vi "Observer.vi"(11 "Name (\"\" to Use UUID)":string) -> ()   [LabVIEW 2025]
uses:
  67f8aefd-9a70-417d-a373-caed4e92e9c8.vi
  acccbc90-5136-4eb0-8ada-bd77d99bf855.vi
  <userlib>/_NEVSTOP/Communicable State Machine(CSM)/AdvanceAPI/CSM - Revert Arguments-Safe String.vi
  <userlib>/_NEVSTOP/Communicable State Machine(CSM)/AdvanceAPI/CSM - Make String Arguments Safe.vi
  <userlib>/_NEVSTOP/Communicable State Machine(CSM)/AdvanceAPI/CSM - Break Down Multiple States String.vi
  <userlib>/_NEVSTOP/Communicable State Machine(CSM)/AdvanceAPI/CSM - Compact Multiple States.vi
  <userlib>/_NEVSTOP/Communicable State Machine(CSM)/AdvanceAPI/CSM - Keywords.vi
  <userlib>/_NEVSTOP/Communicable State Machine(CSM)/_Shared/Trim Single-line Text.vi
  <userlib>/_NEVSTOP/Communicable State Machine(CSM)/_Polymophic/Build Status Broadcast Message.vi
  <userlib>/_NEVSTOP/Communicable State Machine(CSM)/addons/MassData-Parameter/_support/FGV-MassData(lvlibp).vi
  <userlib>/_NEVSTOP/Communicable State Machine(CSM)/_Polymophic/Build Asynchronous Message with Arguments.vi
  <userlib>/_NEVSTOP/Communicable State Machine(CSM)/_Polymophic/Build Synchronous Message with Arguments.vi
  <userlib>/_NEVSTOP/Communicable State Machine(CSM)/Communicable State Machine.lvlib
panel:
  out "Error Occurred":errorcluster
  out "State History":string
  in  "Exit":bool
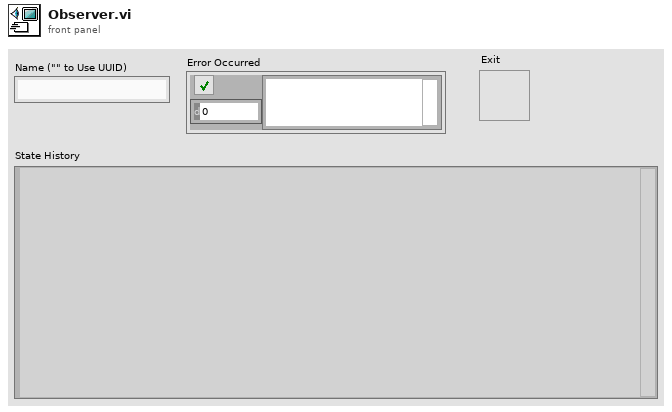
[diagram p1: front panel]
types:
  T1 = enum32{"Invalid", "Standard", "Closed", "Hidden", "Minimized", "Maximized"}
  T2 = enum32{"invalid app kind", "Development System", "Run Time System", "Student Edition", "Embedded LabVIEW", "Evaluation", "Custom"}
  T3 = typedef "Communicable State Machine.lvlib/_CSM_Response Source Message.ctl" = cluster{"‘State":string, "’Arguments":string, "’Error":errorcluster}
  T4 = cluster{"Current VI Reference":refnum<vi>, "Close Panel on Exit?":bool}
  T5 = cluster{"Core":cluster{"Current VI Reference":refnum<vi>, "Close Panel on Exit?":bool}, "player":cluster{"left":i16, "top":i16, "right":i16, "bottom":i16}, "step":i16, "Gate Condition":bool[]}
  T6 = cluster{"left":i16, "top":i16, "right":i16, "bottom":i16}
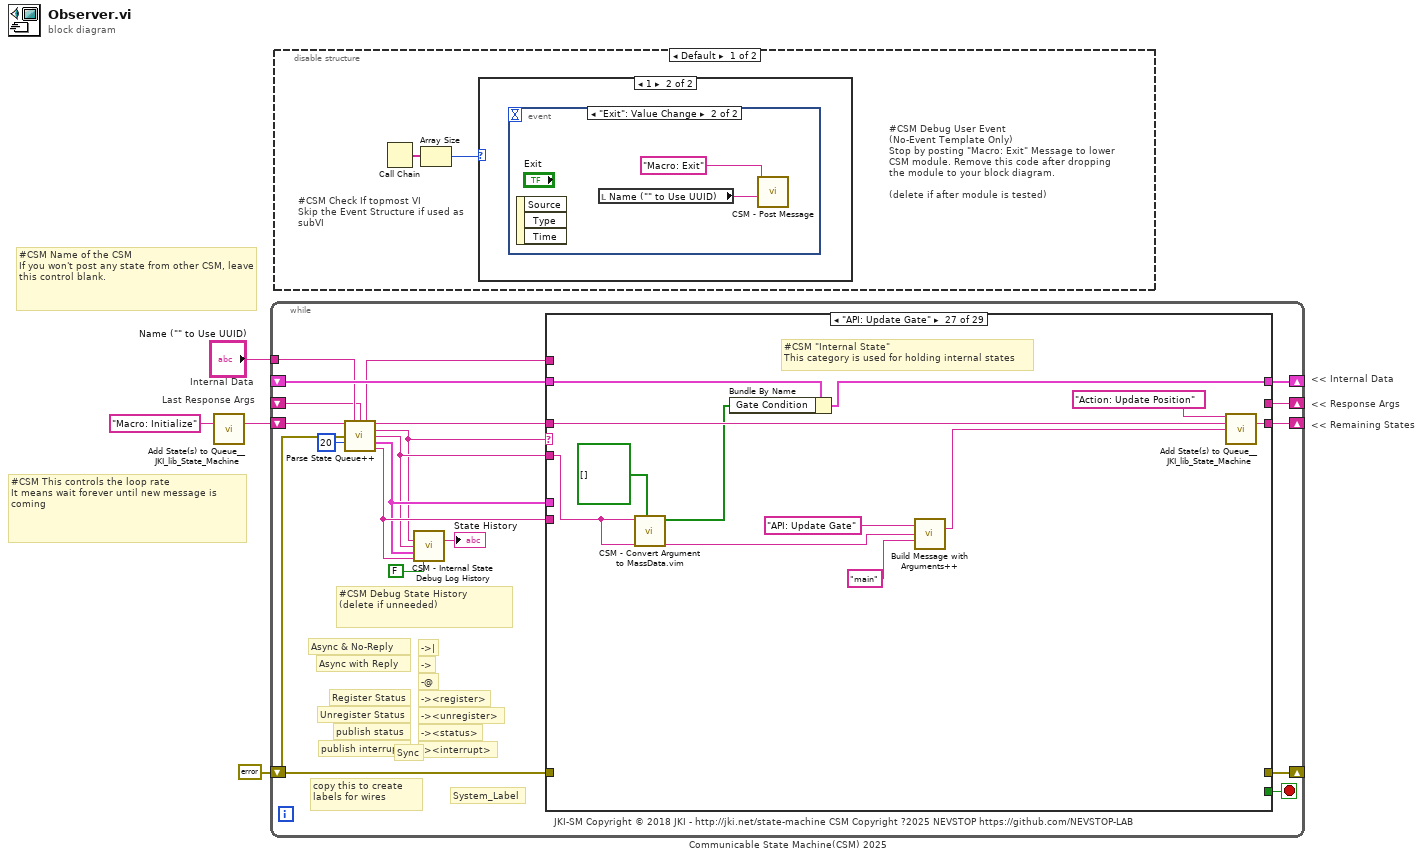
[diagram p0: block diagram]
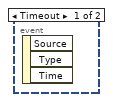
[diagram p3: hidden frame]
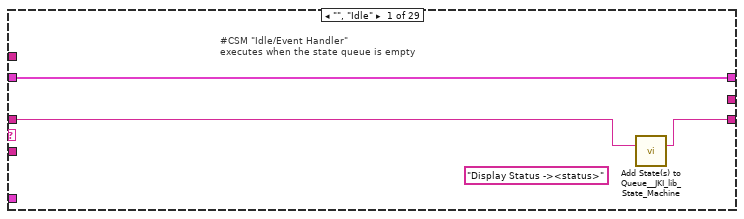
[diagram p5: hidden frame]
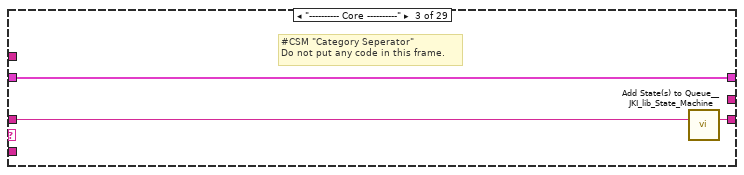
[diagram p7: hidden frame]
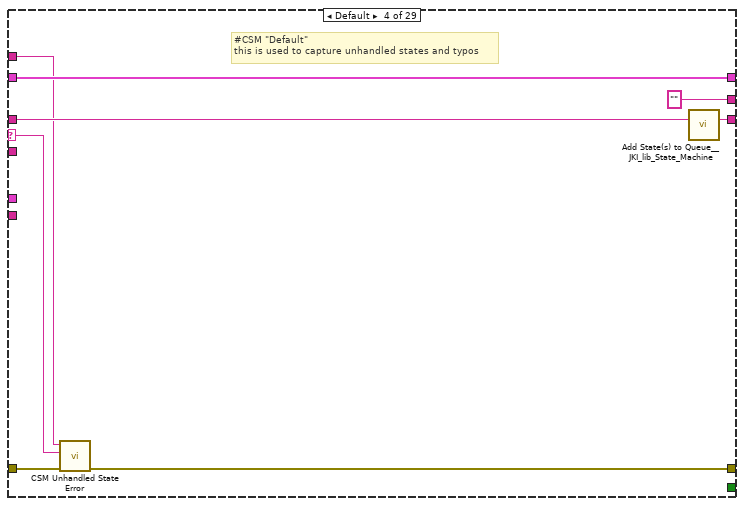
[diagram p8: hidden frame]
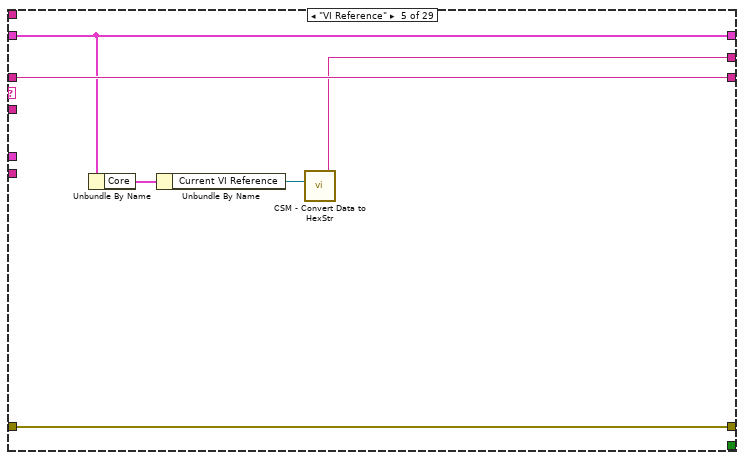
[diagram p9: hidden frame]
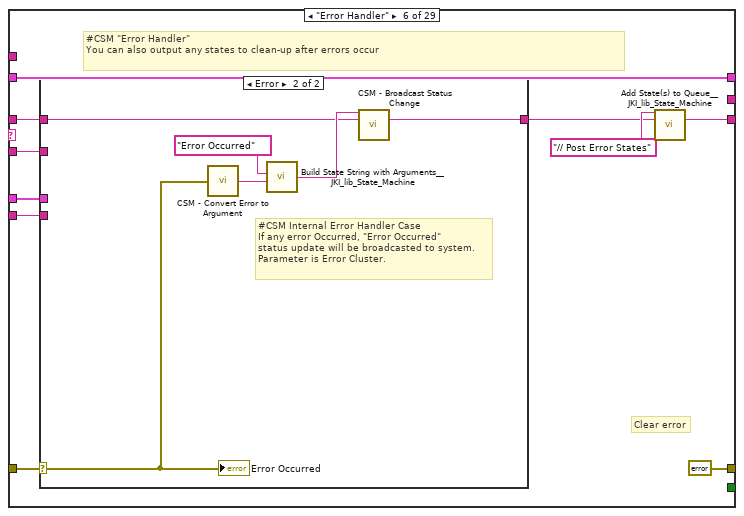
[diagram p10: hidden frame]
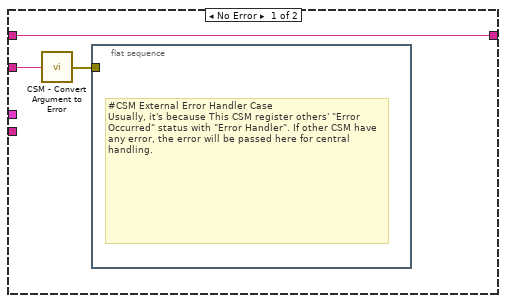
[diagram p11: hidden frame]
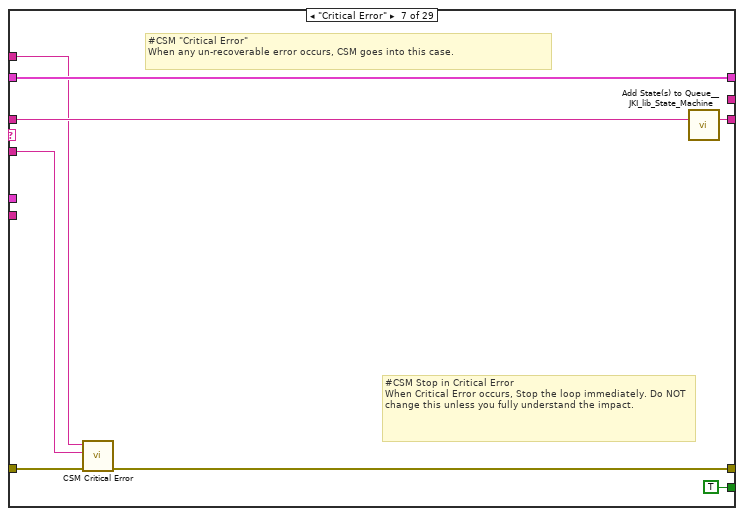
[diagram p12: hidden frame]
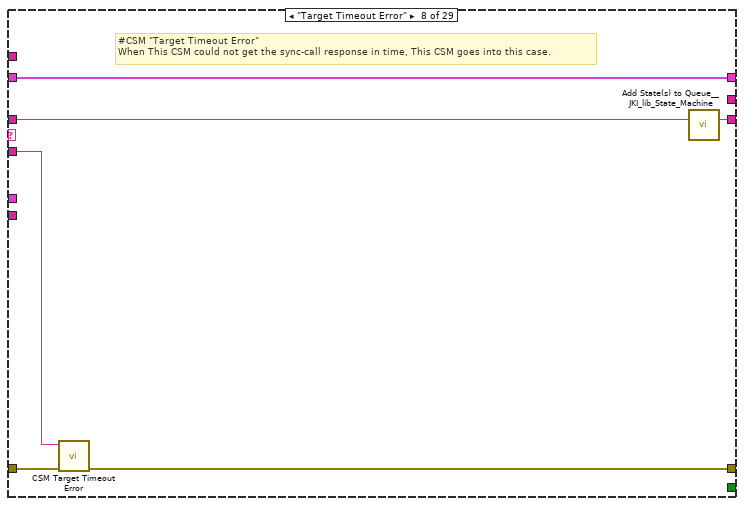
[diagram p13: hidden frame]
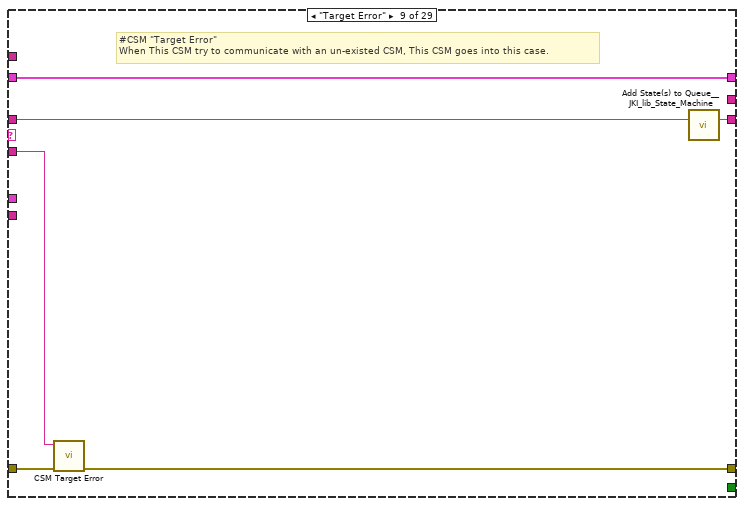
[diagram p14: hidden frame]
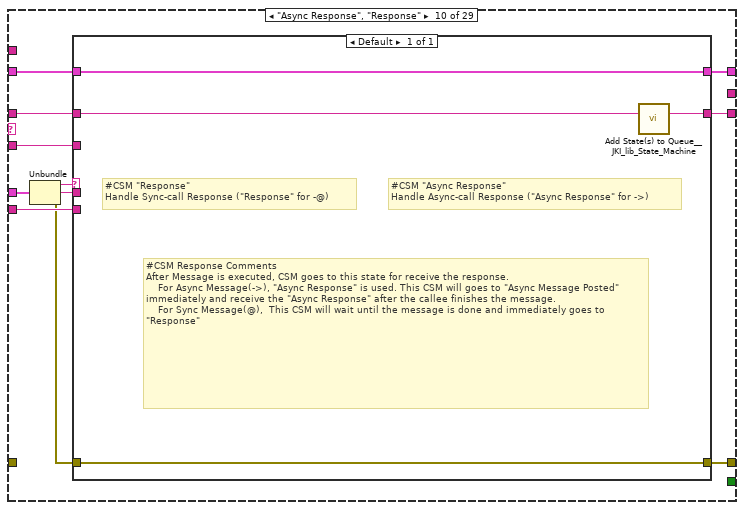
[diagram p15: hidden frame]
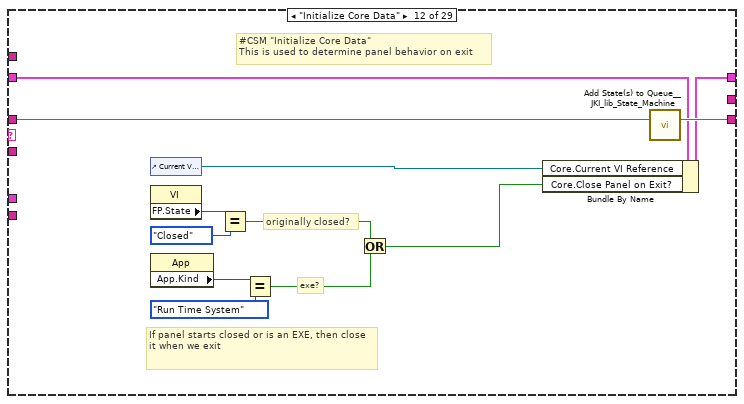
[diagram p17: hidden frame]
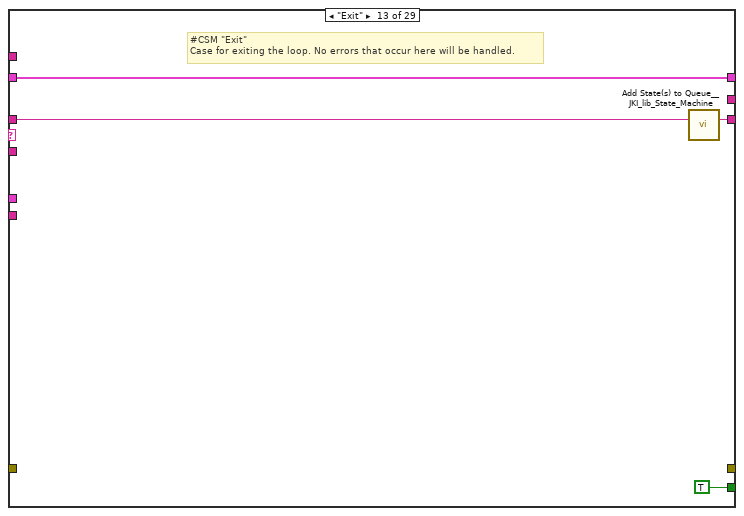
[diagram p18: hidden frame]
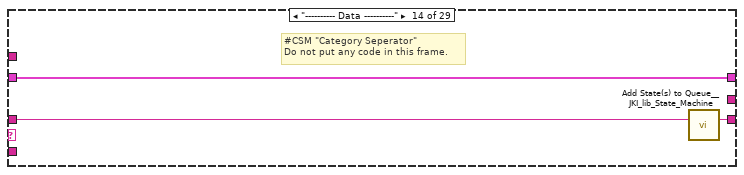
[diagram p19: hidden frame]
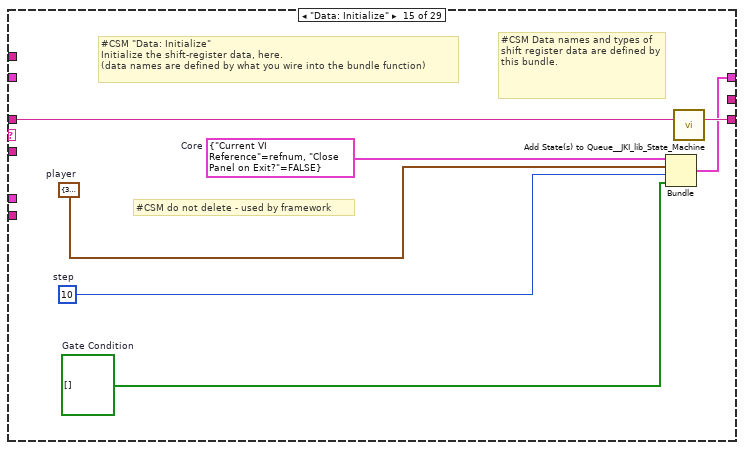
[diagram p20: hidden frame]
diagram:
  # "Last Response Args"
  # "Internal Data"
  # "#CSM Name of the CSM\nIf you won't post any state from other CSM, leave this control blank."
  # "#CSM This controls the loop rate\nIt means wait forever until new message is coming"
  # "<< Internal Data"
  # "<< Response Args"
  # "<< Remaining States"
  n1 = call <vilib>:"Add State(s) to Queue__JKI_lib_State_Machine.vi"("State(s) in (\"\")"="Macro: Initialize" ("Init State(\"Macro: Initialize\")")) -> ("States Out"=w1:string)  [unwired: 14 in]
  n2 = while "Communicable State Machine(CSM) 2025" {
    shift-right: [w18] -> _
    shift-left: _ -> [w17]
    shift-right: [w21] -> _
    shift-left: errorcluster {"status"=FALSE, "code"=0, "source"=""} ("error out") -> [w8]
    shift-right: [w20] -> _
    shift-left: w1 -> [w22]
    tunnel: "Name (\"\" to Use UUID)" -> [w15]
    shift-right: [w16] -> _
    shift-left: _ -> [w10]
    stop <- w19 stop-if-true
    # "#CSM Debug State History\n(delete if unneeded)"
    # "-><interrupt>"
    # "-><status>"
    # "-><unregister>"
    # "-><register>"
    # "-@"
    # "->"
    # "->|"
    # "publish interrupt"
    # "publish status"
    # "Unregister Status"
    # "Register Status"
    # "Sync"
    # "Async with Reply"
    # "Async & No-Reply"
    # "JKI-SM Copyright © 2018 JKI - http://jki.net/state-machine CSM Copyright ?2025 NEVSTOP https://github.com/NEVSTOP-LAB"
    # "copy this to create labels for wires"
    # "System_Label"
    n3 = call <userlib>:"Parse State Queue++.vi"("State Queue"=w22, "Name (\"\" to Use UUID)"=w15, "Response Arguments"=w10, "Previous Error"=w8, "Dequeue (1 ms)"=20) -> ("Name Used"=w9:string, "Remaining States"=w23:string, "Current State"=w11:string, "Arguments"=w12:string, "Additional Information"=w13:T3, "Source CSM"=w14:string)  [unwired: 5 in]
    n4 = call <userlib>:"CSM - Internal State Debug Log History.vi"("State"=w11, "Arguments (\"\")"=w12, ">> Response Source Message >>"=w13, "Source (\"\")"=w14, "Enable Periodic State Filter? (T)"=FALSE) -> ("Debug Log"=→"State History":string)  [unwired: 10 in]
    n5 = case shown="\"API: Update Gate\"" w11 {
      selector: w11 -> [_ _ _ w35 _ _ _ _ _ _ _ _ _ _ _ _ _ _ _ _ _ _ _ _ _ _ _ _ _]
      tunnel: w23 -> [w25 w28 w31 w39 w44 w49 w72 w78 w84 w94 w101 w113 w117 w120 w127 w129 w135 w138 w142 w148 w150 w156 w166 w197 w228 w259 w292 w295 w303]
      tunnel: w12 -> [_ _ _ _ _ w48 w68 w75 w81 w88 _ _ _ _ _ _ _ _ _ _ _ _ _ _ _ _ w283 _ _]
      tunnel: w17 -> [w26 w27 w29 w37 w43 w54 w70 w76 w82 w92 w100 w107 w115 w118 _ w128 w130 w136 w140 w146 w149 w154 w164 w195 w226 w257 w287 w293 w299]
      tunnel: [_ _ _ w32 w45 errorcluster {"status"=FALSE, "code"=0, "source"=""} ("error out") w65 w73 w79 w95 _ _ _ _ _ _ w131 _ _ _ _ w157 _ _ _ _ _ _ _] -> w21
      tunnel: w8 -> [_ _ _ w33 w45 w52 w66 w74 w80 _ _ _ _ _ _ _ w132 _ _ _ _ w157 _ _ _ _ _ _ _]
      tunnel: [w24 w28 w30 w38 w44 w50 w71 w77 w83 w93 w101 w112 w116 w119 w126 w129 w134 w137 w141 w147 w150 w156 w165 w196 w227 w258 w291 w294 w302] -> w20
      tunnel: [_ _ _ _ _ _ TRUE _ _ _ _ _ TRUE _ _ _ _ _ _ _ _ _ _ _ _ _ _ _ _] -> w19
      tunnel: [w26 w27 w29 w37 w43 w54 w70 w76 w82 w91 w100 w111 w115 w118 w125 w128 w130 w136 w140 w146 w149 w153 w163 w194 w225 w256 w286 w293 w299] -> w18
      tunnel: w14 -> [_ _ _ _ _ w47 _ _ _ w89 _ _ _ _ _ _ _ _ _ _ _ _ _ _ _ _ _ _ _]
      tunnel: w13 -> [_ _ _ _ _ w46 _ _ _ w90 _ _ _ _ _ _ _ _ _ _ _ _ _ _ _ _ _ _ _]
      tunnel: [_ _ _ "" w40 _ _ _ _ _ _ _ _ _ _ _ _ _ _ _ _ "Game Reseted" ("HEX String (0-9,A-F)") _ _ _ _ _ _ _] -> w16
      tunnel: w9 -> [_ _ _ w34 _ _ w67 _ _ _ _ _ _ _ _ _ _ _ _ _ _ _ _ _ _ _ _ _ _]
      frame "", "Idle" {
        (unwired) "Display Status -><status>" ("State(s) in Front (\"\")")
        # "#CSM \"Idle/Event Handler\"\nexecutes when the state queue is empty"
        n6 = call <vilib>:"Add State(s) to Queue__JKI_lib_State_Machine.vi"("State(s) in (\"\")"=w25) -> ("States Out"=w24:string)  [unwired: 14 in]
      }
      frame "CSM Documentation" {
        # "#CSM State Syntax\n\n// Comment line, all text to the right of “//” will be ignored\n// Local Message Example\nDoSth: DoA >> Arguments\n\n// Sync Call Example\nAPI: xxxx >> Arguments -@ TargetModule\n\n// Async Call Example\nAPI: xxxx >> Arguments -> TargetModule\n\n// Async Call without Reply Example\nAPI: xxxx >> Arguments ->| TargetModule\n\n// Broadcast normal status:\nStatus >> StatusArguments  -><status>\n\n// Broadcast Interrupt status:\nInterrupt >> StatusArguments  -><interrupt>\n\n// Register Source Module's status to Handler Module\nStatus@Source Module >> Handler Module@Handler Module -><register>\n\n// Unegister Source Module's status\nStatus@Source Module >> Handler Module -><unregister>"
        # "#CSM README FIRST\n\nCommunicable State Machine(CSM) is a LabVIEW application framework that builds upon JKI State Machine(JKISM). It follows the pattern of JKISM and extends the keywords to describe message communication between modules, including concepts such as Sync-Message, Async-Message, Subscription/Unsubscription of status - essential elements for creating reusable code modules. For more information, please visit the CSM wiki: https://nevstop-lab.github.io/CSM-Wiki/\n\nFor instructions on JKI State Machine, visit: \n    http://jki.net/state-machine/\nFor information about CSM, visit: \n    https://github.com/NEVSTOP-LAB"
        # "#CSM \"Documentation\"\nCase for holding CSM Documenation"
      }
      frame "---------- Core ----------" {
        # "#CSM \"Category Seperator\"\nDo not put any code in this frame."
        n7 = call <vilib>:"Add State(s) to Queue__JKI_lib_State_Machine.vi"("State(s) in (\"\")"=w31) -> ("States Out"=w30:string)  [unwired: 14 in]
      }
      frame Default {
        # "#CSM \"Default\"\nthis is used to capture unhandled states and typos"
        n8 = call <userlib>:"CSM Unhandled State Error.vi"("error in (no error)"=w33, "Undefined State"=w35, "CSM Name"=w34) -> ("error out"=w32:errorcluster)  [unwired: 8 in]
        n9 = call <vilib>:"Add State(s) to Queue__JKI_lib_State_Machine.vi"("State(s) in (\"\")"=w39) -> ("States Out"=w38:string)  [unwired: 14 in]
      }
      frame "VI Reference" {
        n10 = Unbundle By Name(w43) -> ("Core"=w42:T4)
        n11 = Unbundle By Name(w42) -> ("Current VI Reference"=w41:refnum<vi>)
        n12 = call <userlib>:"CSM - Convert Data to HexStr.vi"("Variant"=w41) -> ("HEX String (0-9,A-F)"=w40:string)  [unwired: 8 in]
      }
      frame "Error Handler" {
        # "#CSM \"Error Handler\"\nYou can also output any states to clean-up after errors occur"
        # "Clear error"
        n13 = case shown="Error" w52 {
          selector: w52 -> [_ w59]
          tunnel: [w58 w61] -> w51
          tunnel: w49 -> [w58 w60]
          tunnel: w48 -> [w57 _]
          tunnel: w47 -> [_ _]
          tunnel: w46 -> [_ _]
          frame No Error {
            n14 = call <userlib>:"CSM - Convert Argument to Error.vi"("Argument"=w57) -> ("Error"=w56:errorcluster)  [unwired: 4 in]
            n15 = flat-sequence {
              tunnel: w56 -> [_]
              frame #0 {
                # "#CSM External Error Handler Case\nUsually, it's because This CSM register others' \"Error Occurred\" status with \"Error Handler\". If other CSM have any error, the error will be passed here for central handling."
              }
            }
          }
          frame Error {
            # "#CSM Internal Error Handler Case \nIf any error Occurred, \"Error Occurred\" \nstatus update will be broadcasted to system.\nParameter is Error Cluster."
            n16 = call <userlib>:"CSM - Convert Error to Argument.vi"("Error"=w59) -> ("Argument"=w63:string)  [unwired: 4 in]
            n17 = call <vilib>:"Build State String with Arguments__JKI_lib_State_Machine.vi"("Arguments (\"\")"=w63, "State"="Error Occurred" ("Status with Arguments")) -> ("State with Arguments"=w62:string)  [unwired: 4 in]
            n18 = call <userlib>:"CSM - Broadcast Status Change.vi"("Status With Arguments"=w62, "State Queue"=w60) -> ("Remaining States"=w61:string)  [unwired: 13 in]
            "Error Occurred" <- w59
          }
        }
        n19 = call <vilib>:"Add State(s) to Queue__JKI_lib_State_Machine.vi"("State(s) in Front (\"\")"="// Post Error States", "State(s) in (\"\")"=w51) -> ("States Out"=w50:string)  [unwired: 13 in]
      }
      frame "Critical Error" {
        # "#CSM \"Critical Error\"\nWhen any un-recoverable error occurs, CSM goes into this case."
        # "#CSM Stop in Critical Error\nWhen Critical Error occurs, Stop the loop immediately. Do NOT change this unless you fully understand the impact."
        n20 = call <userlib>:"CSM Critical Error.vi"("error in (no error)"=w66, "Arugments (As Reason)"=w68, "CSM Name"=w67) -> ("error out"=w65:errorcluster)  [unwired: 8 in]
        n21 = call <vilib>:"Add State(s) to Queue__JKI_lib_State_Machine.vi"("State(s) in (\"\")"=w72) -> ("States Out"=w71:string)  [unwired: 14 in]
      }
      frame "Target Timeout Error" {
        # "#CSM \"Target Timeout Error\"\nWhen This CSM could not get the sync-call response in time, This CSM goes into this case."
        n22 = call <userlib>:"CSM Target Timeout Error.vi"("error in (no error)"=w74, "Arguments (As CSM Name)"=w75) -> ("error out"=w73:errorcluster)  [unwired: 9 in]
        n23 = call <vilib>:"Add State(s) to Queue__JKI_lib_State_Machine.vi"("State(s) in (\"\")"=w78) -> ("States Out"=w77:string)  [unwired: 14 in]
      }
      frame "Target Error" {
        # "#CSM \"Target Error\"\nWhen This CSM try to communicate with an un-existed CSM, This CSM goes into this case."
        n24 = call <userlib>:"CSM Target Error.vi"("error in (no error)"=w80, "Arguments (As CSM Name)"=w81) -> ("error out"=w79:errorcluster)  [unwired: 9 in]
        n25 = call <vilib>:"Add State(s) to Queue__JKI_lib_State_Machine.vi"("State(s) in (\"\")"=w84) -> ("States Out"=w83:string)  [unwired: 14 in]
      }
      frame "Async Response", "Response" {
        n26 = Unbundle(w90) -> ("‘State"=w87:string, "’Arguments"=w86:string, "’Error"=w85:errorcluster)
        n27 = case shown="Default" w87 {
          tunnel: [w96] -> w93
          tunnel: w94 -> [w97]
          tunnel: [w99] -> w91
          tunnel: w92 -> [w99]
          tunnel: [w98] -> w95
          tunnel: w85 -> [w98]
          tunnel: w89 -> [_]
          tunnel: w88 -> [_]
          tunnel: w86 -> [_]
          frame Default {
            # "#CSM \"Async Response\"\nHandle Async-call Response (\"Async Response\" for ->)"
            # "#CSM \"Response\"\nHandle Sync-call Response (\"Response\" for -@)"
            # "#CSM Response Comments\nAfter Message is executed, CSM goes to this state for receive the response.\n    For Async Message(->), \"Async Response\" is used. This CSM will goes to \"Async Message Posted\" immediately and receive the \"Async Response\" after the callee finishes the message.\n    For Sync Message(@),  This CSM will wait until the message is done and immediately goes to \"Response\""
            n28 = call <vilib>:"Add State(s) to Queue__JKI_lib_State_Machine.vi"("State(s) in (\"\")"=w97) -> ("States Out"=w96:string)  [unwired: 14 in]
          }
        }
      }
      frame "Async Message Posted" {
        # "#CSM \"Async Message Posted\"\nAfter Async Message is posted (-> or ->| ), CSM goes to this state for post-action.\nYou can use Argument - State to tell which Async Message is called."
      }
      frame "Initialize Core Data" {
        # "#CSM \"Initialize Core Data\"\nThis is used to determine panel behavior on exit"
        # "originally closed?"
        # "exe?"
        # "If panel starts closed or is an EXE, then close it when we exit"
        n29 = control-ref of="Current VI Reference"() -> (w105:refnum<vi>)
        n30 = property class="VI"() -> ("FP.State"=w104:T1)  [unwired: 2 in, 2 out]
        n31 = property class="App"() -> ("App.Kind"=w110:T2)  [unwired: 2 in, 2 out]
        n32 = Equal?(x=w104, y=T1."Closed" ("Front Panel Window:State")) -> (x = y?=w102:bool)
        n33 = Equal?(x=w110, y=T2."Run Time System" ("Application:Kind")) -> (x = y?=w108:bool)
        n34 = Or(x=w102, y=w108) -> (x .or. y?=w106:bool)
        n35 = Bundle By Name(cluster=w107, "Core.Current VI Reference"=w105, "Core.Close Panel on Exit?"=w106) -> (w111:T5)
        n36 = call <vilib>:"Add State(s) to Queue__JKI_lib_State_Machine.vi"("State(s) in (\"\")"=w113) -> ("States Out"=w112:string)  [unwired: 14 in]
      }
      frame "Exit" {
        # "#CSM \"Exit\"\nCase for exiting the loop. No errors that occur here will be handled."
        n37 = call <vilib>:"Add State(s) to Queue__JKI_lib_State_Machine.vi"("State(s) in (\"\")"=w117) -> ("States Out"=w116:string)  [unwired: 14 in]
      }
      frame "---------- Data ----------" {
        # "#CSM \"Category Seperator\"\nDo not put any code in this frame."
        n38 = call <vilib>:"Add State(s) to Queue__JKI_lib_State_Machine.vi"("State(s) in (\"\")"=w120) -> ("States Out"=w119:string)  [unwired: 14 in]
      }
      frame "Data: Initialize" {
        w121 = bool[] []  # Gate Condition
        w122 = i16 10  # step
        w123 = T6 {"left"=375, "top"=375, "right"=425, "bottom"=425}  # player
        w124 = T4 {"Current VI Reference"=refnum, "Close Panel on Exit?"=FALSE}  # Core
        # "#CSM \"Data: Initialize\"\nInitialize the shift-register data, here.\n(data names are defined by what you wire into the bundle function)"
        # "#CSM do not delete - used by framework"
        # "#CSM Data names and types of shift register data are defined by this bundle."
        n39 = Bundle("Core"=w124, "player"=w123, "step"=w122, "Gate Condition"=w121) -> (w125:T5)  [unwired: 1 in]
        n40 = call <vilib>:"Add State(s) to Queue__JKI_lib_State_Machine.vi"("State(s) in (\"\")"=w127) -> ("States Out"=w126:string)  [unwired: 14 in]
      }
      frame "Data: Update Indicators" {
      }
      frame "Data: Cleanup" {
        # "#CSM \"Data: Cleanup\"\nCleanup any data and references, here.\n(this is called automatically, by the Macro: Exit)"
        n41 = Unbundle By Name(w130) -> ("Core.Current VI Reference"=w133:refnum<vi>)
        n42 = Close Reference(reference=w133, error in (no error)=w132) -> (error out=w131:errorcluster)
        n43 = call <vilib>:"Add State(s) to Queue__JKI_lib_State_Machine.vi"("State(s) in (\"\")"=w135) -> ("States Out"=w134:string)  [unwired: 14 in]
      }
      frame "---------- Macro ----------" {
        # "#CSM \"Category Seperator\"\nDo not put any code in this frame."
        n44 = call <vilib>:"Add State(s) to Queue__JKI_lib_State_Machine.vi"("State(s) in (\"\")"=w138) -> ("States Out"=w137:string)  [unwired: 14 in]
      }
      frame "Macro: Initialize" {
        # "#CSM \"Macro: Initialize\"\nInitialization Macro (This is called once, when the VI starts)"
        n45 = call <vilib>:"Add State(s) to Queue__JKI_lib_State_Machine.vi"("State(s) in Front (\"\")"="Initialize Core Data\nData: Initialize\nData: Update Indicators", "State(s) in (\"\")"=w142) -> ("States Out"=w141:string)  [unwired: 13 in]
      }
      frame "Macro: Exit" {
        # "#CSM \"Macro: Exit\"\nExit Macro (This is called once, when the VI exits)"
        n46 = call <vilib>:"Add State(s) to Queue__JKI_lib_State_Machine.vi"("State(s) in Front (\"\")"="//Exit Sub-Modules ", "State(s) at Back (\"\")"="Data: Cleanup\nExit") -> ("States Out"=w144:string)  [unwired: 13 in]
        n47 = call <vilib>:"Add State(s) to Queue__JKI_lib_State_Machine.vi"("State(s) in Front (\"\")"=w144, "State(s) in (\"\")"=w148) -> ("States Out"=w147:string)  [unwired: 13 in]
      }
      frame "---------- API ----------" {
        # "#CSM \"Category Seperator\"\nDo not put any code in this frame."
      }
      frame "API: Reset Game" {
        w151 = bool[] [FALSE, FALSE, FALSE, FALSE]  # Gate Condition
        w152 = T6 {"left"=375, "top"=375, "right"=425, "bottom"=425}  # player
        n48 = Bundle By Name(cluster=w154, "player"=w152, "Gate Condition"=w151) -> (w153:T5)
      }
      frame "API: Move Up" {
        # "#CSM API Example\nCopy/Rename this case for your own API"
        n49 = Unbundle By Name(w164) -> ("player.top"=w159:i16, "player.bottom"=w161:i16, "step"=w162:i16)
        n50 = Less Or Equal?(x=w159, y=i16 0) -> (x <= y?=w160:bool)
        n51 = case shown="True" w160 {
          tunnel: w166 -> [w175 w186]
          tunnel: [w174 w187] -> w165
          tunnel: w164 -> [w173 w183]
          tunnel: [w172 w182] -> w163
          tunnel: w162 -> [w169 _]
          tunnel: w161 -> [w171 w180]
          tunnel: w159 -> [w168 w181]
          frame False {
            n52 = Subtract(x=w171, y=w169) -> (x-y=w170:i16)
            n53 = Subtract(x=w168, y=w169) -> (x-y=w167:i16)
            n54 = Bundle By Name(cluster=w173, "player.top"=w167, "player.bottom"=w170) -> (w172:T5)
            n55 = call <vilib>:"Add State(s) to Queue__JKI_lib_State_Machine.vi"("State(s) in (\"\")"=w175, "State(s) at Back (\"\")"="Action: Update Position" ("State(s) at Back (\"\")")) -> ("States Out"=w174:string)  [unwired: 13 in]
          }
          frame True {
            w179 = i16 750 ("y")
            n56 = Add(x=w180, y=w179) -> (x+y=w178:i16)
            n57 = Add(x=w181, y=w179) -> (x+y=w177:i16)
            n58 = Bundle By Name(cluster=w183, "player.top"=w177, "player.bottom"=w178) -> (w182:T5)
            n59 = call-poly <userlib>:"Build Message with Arguments++.vi"("State With Arguments"="Switch Room", "Arguments (\"\")"="Gate Up" ("Arguments (\"\")")) -> ("CSM Message String"=w185:string)  [unwired: 13 in]
            n60 = call <vilib>:"Add State(s) to Queue__JKI_lib_State_Machine.vi"("State(s) in (\"\")"=w186, "State(s) at Back (\"\")"=w185) -> ("States Out"=w187:string)  [unwired: 13 in]
          }
        }
      }
      frame "API: Move Down" {
        # "#CSM API Example\nCopy/Rename this case for your own API"
        n61 = Unbundle By Name(w195) -> ("player.top"=w192:i16, "player.bottom"=w190:i16, "step"=w193:i16)
        n62 = Greater Or Equal?(x=w190, y=i16 800) -> (x >= y?=w191:bool)
        n63 = case shown="True" w191 {
          tunnel: w197 -> [w206 w217]
          tunnel: [w205 w218] -> w196
          tunnel: w195 -> [w204 w214]
          tunnel: [w203 w213] -> w194
          tunnel: w193 -> [w198 _]
          tunnel: w190 -> [w201 w211]
          tunnel: w192 -> [w199 w212]
          frame False {
            n64 = Add(x=w201, y=w198) -> (x+y=w202:i16)
            n65 = Add(x=w199, y=w198) -> (x+y=w200:i16)
            n66 = Bundle By Name(cluster=w204, "player.top"=w200, "player.bottom"=w202) -> (w203:T5)
            n67 = call <vilib>:"Add State(s) to Queue__JKI_lib_State_Machine.vi"("State(s) in (\"\")"=w206, "State(s) at Back (\"\")"="Action: Update Position" ("State(s) at Back (\"\")")) -> ("States Out"=w205:string)  [unwired: 13 in]
          }
          frame True {
            w208 = i16 750 ("y")
            n68 = Subtract(x=w211, y=w208) -> (x-y=w209:i16)
            n69 = Subtract(x=w212, y=w208) -> (x-y=w210:i16)
            n70 = Bundle By Name(cluster=w214, "player.top"=w210, "player.bottom"=w209) -> (w213:T5)
            n71 = call-poly <userlib>:"Build Message with Arguments++.vi"("State With Arguments"="Switch Room", "Arguments (\"\")"="Gate Down" ("Arguments (\"\")")) -> ("CSM Message String"=w216:string)  [unwired: 13 in]
            n72 = call <vilib>:"Add State(s) to Queue__JKI_lib_State_Machine.vi"("State(s) in (\"\")"=w217, "State(s) at Back (\"\")"=w216) -> ("States Out"=w218:string)  [unwired: 13 in]
          }
        }
      }
      frame "API: Move Left" {
        # "#CSM API Example\nCopy/Rename this case for your own API"
        n73 = Unbundle By Name(w226) -> ("player.left"=w221:i16, "player.right"=w223:i16, "step"=w224:i16)
        n74 = Less Or Equal?(x=w221, y=i16 0) -> (x <= y?=w222:bool)
        n75 = case shown="True" w222 {
          tunnel: w228 -> [w237 w248]
          tunnel: [w236 w249] -> w227
          tunnel: w226 -> [w235 w245]
          tunnel: [w234 w244] -> w225
          tunnel: w224 -> [w229 _]
          tunnel: w223 -> [w233 w242]
          tunnel: w221 -> [w230 w243]
          frame False {
            n76 = Subtract(x=w233, y=w229) -> (x-y=w232:i16)
            n77 = Subtract(x=w230, y=w229) -> (x-y=w231:i16)
            n78 = Bundle By Name(cluster=w235, "player.left"=w231, "player.right"=w232) -> (w234:T5)
            n79 = call <vilib>:"Add State(s) to Queue__JKI_lib_State_Machine.vi"("State(s) in (\"\")"=w237, "State(s) at Back (\"\")"="Action: Update Position" ("State(s) at Back (\"\")")) -> ("States Out"=w236:string)  [unwired: 13 in]
          }
          frame True {
            w241 = i16 750 ("y")
            n80 = Add(x=w242, y=w241) -> (x+y=w239:i16)
            n81 = Add(x=w243, y=w241) -> (x+y=w240:i16)
            n82 = Bundle By Name(cluster=w245, "player.left"=w240, "player.right"=w239) -> (w244:T5)
            n83 = call-poly <userlib>:"Build Message with Arguments++.vi"("State With Arguments"="Switch Room", "Arguments (\"\")"="Gate Left" ("Arguments (\"\")")) -> ("CSM Message String"=w247:string)  [unwired: 13 in]
            n84 = call <vilib>:"Add State(s) to Queue__JKI_lib_State_Machine.vi"("State(s) in (\"\")"=w248, "State(s) at Back (\"\")"=w247) -> ("States Out"=w249:string)  [unwired: 13 in]
          }
        }
      }
      frame "API: Move Right" {
        # "#CSM API Example\nCopy/Rename this case for your own API"
        n85 = Unbundle By Name(w257) -> ("player.left"=w254:i16, "player.right"=w253:i16, "step"=w255:i16)
        n86 = Greater Or Equal?(x=w253, y=i16 800) -> (x >= y?=w252:bool)
        n87 = case shown="True" w252 {
          tunnel: w259 -> [w268 w279]
          tunnel: [w267 w280] -> w258
          tunnel: w257 -> [w266 w276]
          tunnel: [w265 w275] -> w256
          tunnel: w255 -> [w260 _]
          tunnel: w253 -> [w263 w273]
          tunnel: w254 -> [w261 w274]
          frame False {
            n88 = Add(x=w263, y=w260) -> (x+y=w264:i16)
            n89 = Add(x=w261, y=w260) -> (x+y=w262:i16)
            n90 = Bundle By Name(cluster=w266, "player.left"=w262, "player.right"=w264) -> (w265:T5)
            n91 = call <vilib>:"Add State(s) to Queue__JKI_lib_State_Machine.vi"("State(s) in (\"\")"=w268, "State(s) at Back (\"\")"="Action: Update Position" ("State(s) at Back (\"\")")) -> ("States Out"=w267:string)  [unwired: 13 in]
          }
          frame True {
            w270 = i16 750 ("y")
            n92 = Subtract(x=w273, y=w270) -> (x-y=w271:i16)
            n93 = Subtract(x=w274, y=w270) -> (x-y=w272:i16)
            n94 = Bundle By Name(cluster=w276, "player.left"=w272, "player.right"=w271) -> (w275:T5)
            n95 = call-poly <userlib>:"Build Message with Arguments++.vi"("State With Arguments"="Switch Room", "Arguments (\"\")"="Gate Right" ("Arguments (\"\")")) -> ("CSM Message String"=w278:string)  [unwired: 13 in]
            n96 = call <vilib>:"Add State(s) to Queue__JKI_lib_State_Machine.vi"("State(s) in (\"\")"=w279, "State(s) at Back (\"\")"=w278) -> ("States Out"=w280:string)  [unwired: 13 in]
          }
        }
      }
      frame "API: Update Gate" {
        # "#CSM \"Internal State\"\nThis category is used for holding internal states"
        n97 = call "CSM - Convert Argument to MassData.vim"("Type"=bool[] [] ("Gate Condition"), "MassData Argument"=w283) -> ("Data"=w284:bool[])  [unwired: 6 in, 1 out]
        n98 = Bundle By Name(cluster=w287, "Gate Condition"=w284) -> (w286:T5)
        n99 = call-poly <userlib>:"Build Message with Arguments++.vi"("State With Arguments"="API: Update Gate", "Arguments (\"\")"=w283, "Target Module (\"\")"="main" ("Target Module (\"\")")) -> ("CSM Message String"=w288:string)  [unwired: 12 in]
        n100 = call <vilib>:"Add State(s) to Queue__JKI_lib_State_Machine.vi"("State(s) in Front (\"\")"="Action: Update Position" ("State(s) in Front (\"\")"), "State(s) in (\"\")"=w292, "State(s) at Back (\"\")"=w288) -> ("States Out"=w291:string)  [unwired: 12 in]
      }
      frame "---------- Action ----------" {
        # "#CSM \"Category Seperator\"\nDo not put any code in this frame."
        n101 = call <vilib>:"Add State(s) to Queue__JKI_lib_State_Machine.vi"("State(s) in (\"\")"=w295) -> ("States Out"=w294:string)  [unwired: 14 in]
      }
      frame "Action: Update Position" {
        # "#CSM \"Internal State\"\nThis category is used for holding internal states"
        n102 = Unbundle By Name(w299) -> ("player"=w298:T6)
        n103 = call "CSM - Convert MassData to Argument.vim"("Data"=w298) -> ("MassData Argument"=w297:string)  [unwired: 7 in, 1 out]
        n104 = call-poly <userlib>:"Build Message with Arguments++.vi"("State With Arguments"="API: Update Position", "Arguments (\"\")"=w297, "Target Module (\"\")"="main" ("Target Module (\"\")")) -> ("CSM Message String"=w296:string)  [unwired: 12 in]
        n105 = call <vilib>:"Add State(s) to Queue__JKI_lib_State_Machine.vi"("State(s) in (\"\")"=w303, "State(s) at Back (\"\")"=w296) -> ("States Out"=w302:string)  [unwired: 13 in]
      }
    }
  }
  n106 = disable-structure shown="Default" {
    frame condition #0 (active) {
      # "#CSM Check If topmost VI\nSkip the Event Structure if used as subVI"
      # "#CSM Debug User Event\n(No-Event Template Only)\nStop by posting \"Macro: Exit\" Message to lower CSM module. Remove this code after dropping the module to your block diagram. \n\n(delete if after module is tested)"
      n107 = Call Chain() -> (call chain=w305:string[])
      n108 = Array Size(array=w305) -> (size(s)=w304:i32)
      n109 = case shown="1" w304 {
        frame Default {
        }
        frame 1 {
          n110 = event shown="[1] \"Exit\": Value Change" {
            selector: _ -> [_ _]
            dyn-events: _ -> [_ _]
            timeout: _ -> [_ _]
            event Timeout {
              n111 = event-data() -> ()  [unwired: 1 in, 3 out]
            }
            event "Exit": Value Change {
              n112 = event-data() -> ()  [unwired: 1 in, 3 out]
              n113 = local read "Name (\"\" to Use UUID)"() -> (w307:string)
              n114 = call <userlib>:"CSM - Post Message.vi"("Target Module"=w307, "State"="Macro: Exit" ("States")) -> ()  [unwired: 9 in, 1 out]
            }
          }
        }
      }
    }
    frame condition #1 {
    }
  }
